vi "Response Message.vi"(8 "error in (no error)":errorcluster, 9 "Response Message Data":variant, 10 "Response Message":string, 11 "Process In":refnum<class "Process.lvclass">) -> (0 "error out":errorcluster, 3 "Process Out":refnum<class "Process.lvclass">)   [LabVIEW 2020, in "Process.lvclass"]
doc: "Respond to a request message. The response will only be delivered to the requesting method and. \nThis VI may only be called from within the same case of the Handle Messages VI which handles the request or from a Helper Loop or Asynchronous Action launched from the specific case."
uses:
  Process.lvclass
  C:/git/astemes-triarc-framework/source/Framework/Logging/Logging.lvclass
  Process.lvclass/Process.ctl
  Logging/Log Debug.vi
  <vilib>/AdvancedString/1D String Array to Delimited String.vi
  <vilib>/Utility/High Resolution Relative Seconds.vi
  <vilib>/Utility/error.llb/Error Cluster From Error Code.vi
  Public/Read Name.vi
  <vilib>/ErrorRing/Error Ring.xnode
  Callback/Callback.lvclass
  Logging/Logging.lvclass
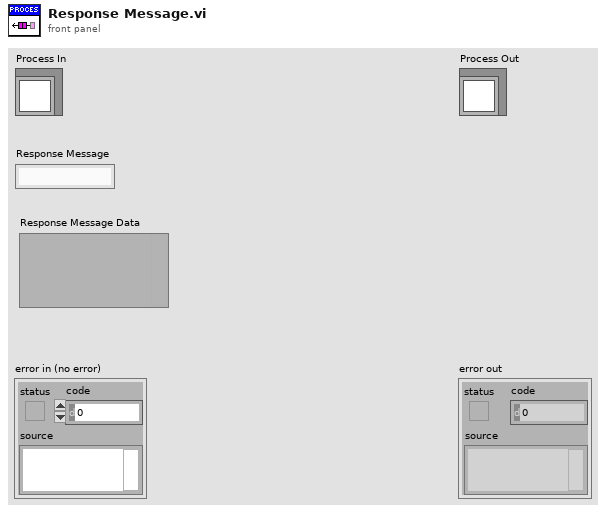
[diagram p1: front panel]
types:
  T1 = typedef "Process.lvclass/API Mode.ctl" = enum16{"Send Message", "Handle Message"}
  T2 = typedef "Process.lvclass/Lifecycle State.ctl" = enum16{"Uninitialized", "Initialized", "Started", "Running", "Stopped", "Finished"}
  T3 = enum16{"Send", "Receive", "Request", "Response", "Broadcast"}
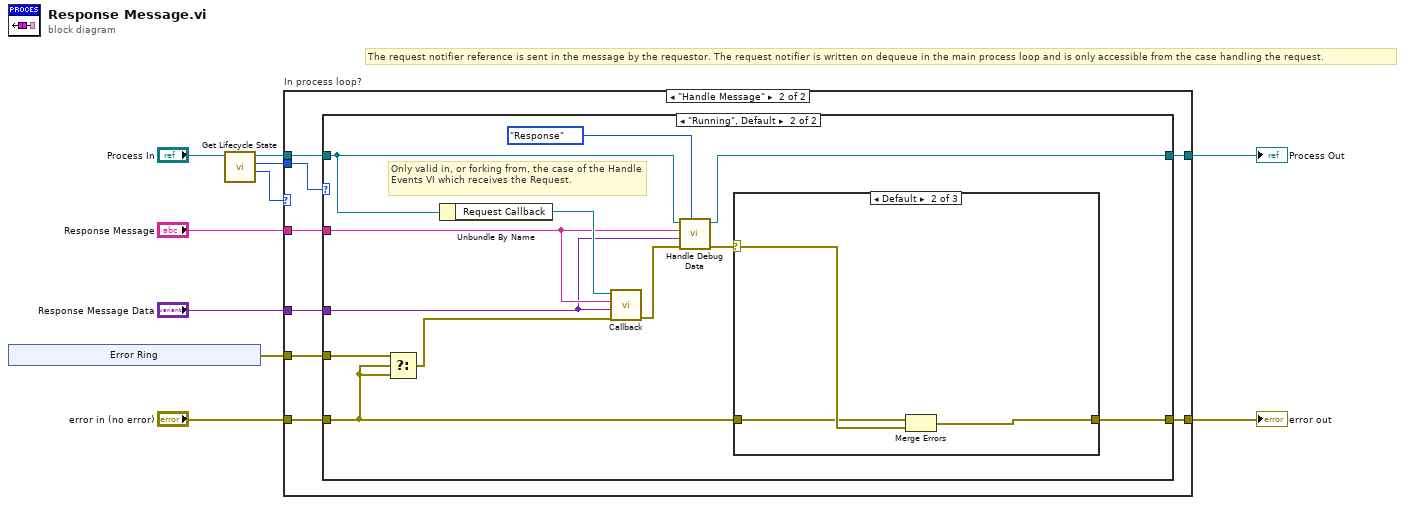
[diagram p0: block diagram]
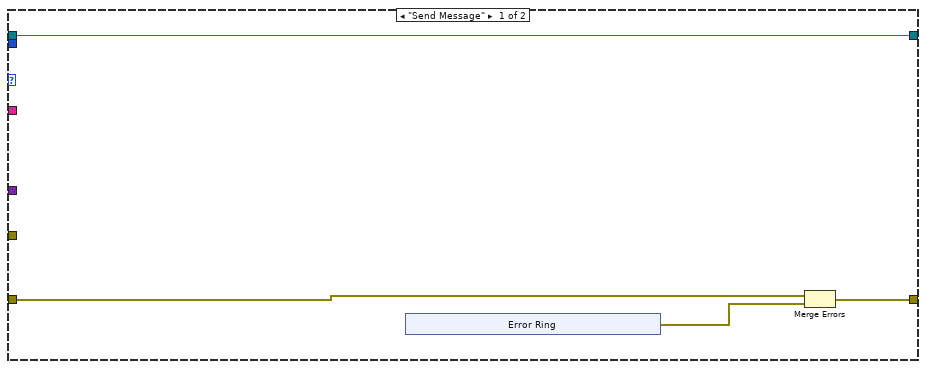
[diagram p2: hidden frame]
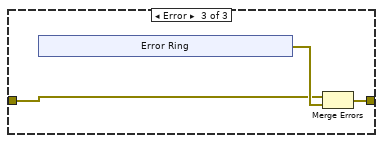
[diagram p5: hidden frame]
diagram:
  # "The request notifier reference is sent in the message by the requestor. The request notifier is written on dequeue in the main process loop and is only accessible from the case handling the request."
  n1 = xnode "Error Ring"() -> ("error out"=w1:errorcluster)
  n2 = call "Get Lifecycle State.vi"("Process In"="Process In") -> ("API Mode"=w2:T1, "Lifecycle State"=w3:T2, "Process Out"=w4:refnum<class "Process.lvclass">)  [unwired: 7 in, 1 out]
  n3 = case "In process loop?" shown="\"Handle Message\"" w2 {
    tunnel: "Response Message" -> [_ w26]
    tunnel: "Response Message Data" -> [_ w25]
    tunnel: [w13 w24] -> w6
    tunnel: w4 -> [w14 w23]
    tunnel: "error in (no error)" -> [w12 w22]
    tunnel: w3 -> [_ w21]
    tunnel: [w14 w20] -> w5
    tunnel: w1 -> [_ w19]
    frame "Send Message" {
      n4 = xnode "Error Ring"() -> ("error out"=w11:errorcluster)
      n5 = Merge Errors(w12, w11) -> (w13:errorcluster)
    }
    frame "Handle Message" {
      n6 = case shown="\"Running\", Default" w21 {
        tunnel: w26 -> [_ w31]
        tunnel: w25 -> [_ w30]
        tunnel: [w27 w38] -> w24
        tunnel: w23 -> [w28 w35]
        tunnel: w22 -> [w27 w34]
        tunnel: [w28 w36] -> w20
        tunnel: w19 -> [_ w33]
        frame "Stopped" {
          # "If the process is stopped, the wait for reply VI will abort and throw an error. \nThere is no reason to throw an error here as well."
        }
        frame "Running", Default {
          # "Only valid in, or forking from, the case of the Handle Events VI which receives the Request."
          n7 = Select(t=w33, s=w34, f=w34) -> (s? t:f=w29:errorcluster)
          n8 = Unbundle By Name(w35) -> ("Request Callback"=w40:refnum<class "Callback.lvclass">)
          n9 = call-dynamic "Callback.vi"("error in (no error)"=w29, "Message Data"=w30, "Message"=w31, "Callback in"=w40) -> ("error out"=w39:errorcluster)  [unwired: 7 in]
          n10 = call "Handle Debug Data.vi"("Action"=T3."Response", "error in (no error)"=w39, "Message Data"=w30, "Message"=w31, "Process In"=w35) -> ("error out"=w37:errorcluster, "Process Out"=w36:refnum<class "Process.lvclass">)  [unwired: 5 in]
          n11 = case shown="Default" w37 {
            selector: w37 -> [_ w44 _]
            tunnel: [w41 w43 w46] -> w38
            tunnel: w34 -> [w41 w42 w45]
            frame No Error {
            }
            frame Default {
              n12 = Merge Errors(w42, w44) -> (w43:errorcluster)
            }
            frame Error {
              n13 = xnode "Error Ring"() -> ("error out"=w47:errorcluster)
              n14 = Merge Errors(w45, w47) -> (w46:errorcluster)
            }
          }
        }
      }
    }
  }
  "error out" <- w6
  "Process Out" <- w5
